vi "DCC Get Multi Parameters.vi"(8 "Error In":errorcluster, 10 "Module No":i16, 11 "DLL Path":path) -> (0 "Error Out":errorcluster, 2 "Module No":i16, 3 "DLL Path":path, 4 "Data Cluster":T1)   [LabVIEW 2019]
doc: "After calling the Initialize VI the measurement parameters from the initialisation file are present in the module and in the internal data structures of the DLLs.\nFor reading these parameters the \"DCC_get_parameters\"will be used.\nThis function transfers the parameter values of the DCC module specified by the module number.\n\nOctober 2018\nFrank Quadt & Stefan Smietana\ninfo@becker-hickl.com"
uses:
  DCC_Controls/DCC_Data_Cluster.ctl
panel:
  # "(c) 2021 Becker & Hickl GmbH\n     All Rights Reserved."
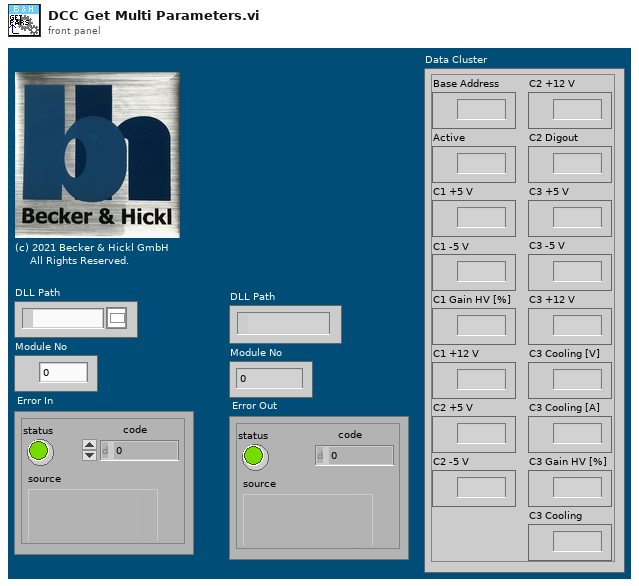
[diagram p1: front panel]
types:
  T1 = typedef "DCC_Data_Cluster.ctl" = cluster{"Base Address":u16, "Active":i16, "C1 +5 V":i16, "C1 -5 V":i16, "C1 Gain HV [%]":sgl, "C1 +12 V":i16, "C2 +5 V":i16, "C2 -5 V":i16, "C2 +12 V":i16, "C2 Digout":i16, "C3 +5 V":i16, "C3 -5 V":i16, "C3 +12 V":i16, "C3 Cooling [V]":sgl, "C3 Cooling [A]":sgl, "C3 Gain HV [%]":sgl, "C3 Cooling":i16}
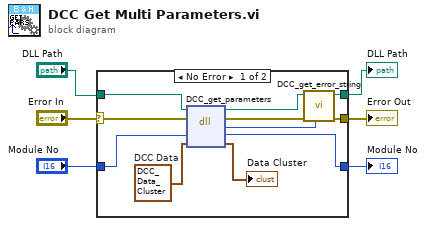
[diagram p0: block diagram]
diagram:
  n1 = case shown="No Error" "Error In" {
    selector: "Error In" -> [w17 w19]
    tunnel: [w13 w19] -> w5
    tunnel: [w12 w20] -> w4
    tunnel: "DLL Path" -> [w16 w20]
    tunnel: "Module No" -> [w11 w18]
    tunnel: [w9 w18] -> w1
    frame No Error {
      w8 = T1 {"Base Address"=0, "Active"=0, "C1 +5 V"=0, "C1 -5 V"=0, "C1 Gain HV [%]"=0.0, "C1 +12 V"=0, "C2 +5 V"=0, "C2 -5 V"=0, "C2 +12 V"=0, "C2 Digout"=0, "C3 +5 V"=0, "C3 -5 V"=0, "C3 +12 V"=0, "C3 Cooling [V]"=0.0, "C3 Cooling [A]"=0.0, "C3 Gain HV [%]"=0.0, "C3 Cooling"=0}  # DCC Data
      n2 = dll-call lib="C:/Program Files (x86)/BH/DCC/DLL/dcc64.dll" fn="DCC_get_parameters"(path in=w16, error in=w17, "ModuleNo"=w11, "DataCluster"=w8) -> (path out=w15:path, error out=w14:errorcluster, "return type"=w10:i16, "ModuleNo"=w9:i16, "DataCluster"=→"Data Cluster":T1)  [unwired: 1 in]
      n3 = call "DCC_get_error_string.vi"("Error ID"=w10, "Error In"=w14, "DLL Path"=w15) -> ("Error Out"=w13:errorcluster, "DLL Path"=w12:path)  [unwired: 6 in, 1 out]
    }
    frame Error {
    }
  }
  "Error Out" <- w5
  "DLL Path" <- w4
  "Module No" <- w1
